vi "Read Parent UID.vi"(8 "error in (no error)":errorcluster, 11 "Generic Node in":refnum<class "Generic Node.lvclass">) -> (0 "error out":errorcluster, 2 "Parent UID":string, 3 "Generic Node out":refnum<class "Generic Node.lvclass">)   [LabVIEW 2017, in "opcua.lvlib" / "Browser Core.lvlib" / "Generic Node.lvclass"]
uses:
  Generic Node.lvclass
  Generic Node.lvclass/Generic Node.ctl
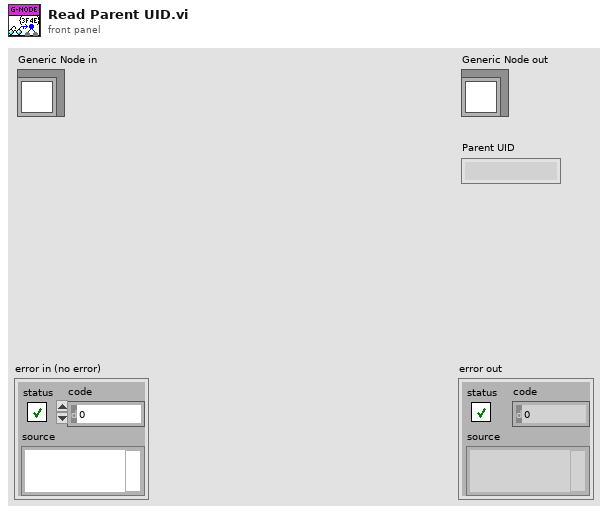
[diagram p1: front panel]
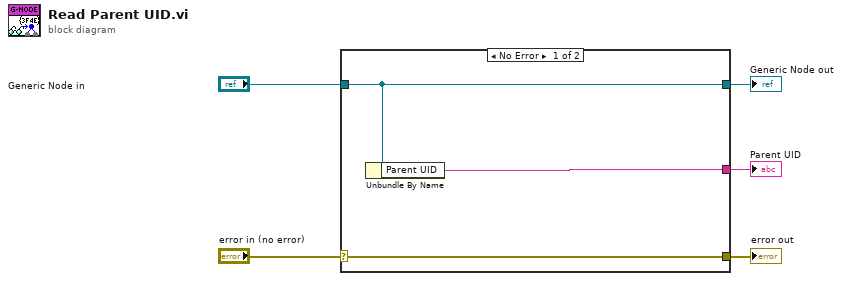
[diagram p0: block diagram]
diagram:
  n1 = case shown="No Error" "error in (no error)" {
    selector: "error in (no error)" -> [w8 w9]
    tunnel: [w8 w9] -> w4
    tunnel: [w7 w10] -> w2
    tunnel: "Generic Node in" -> [w7 w10]
    tunnel: [w6 _] -> w1
    frame No Error {
      n2 = Unbundle By Name(w7) -> ("Parent UID"=w6:string)
    }
    frame Error {
    }
  }
  "error out" <- w4
  "Generic Node out" <- w2
  "Parent UID" <- w1
